vi "Set Alarm Colors and Get Alarm Text.vi"(9 "Alarm reference":refnum<vi>, 10 "Under Low Limit":bool, 11 "Over High Limit":bool) -> (3 "Alarm String":string)   [LabVIEW 2023]
doc: "Sets the colors of the Alarm display based on the alarm state and returns the text to display in the Alarm indicator."
uses:
  <vilib>/Utility/miscctls.llb/LVTextColorsTypeDef.ctl
panel:
  in  "Under Temp":string="UNDER TEMP"
  in  "Over Temp":string="OVER TEMP"
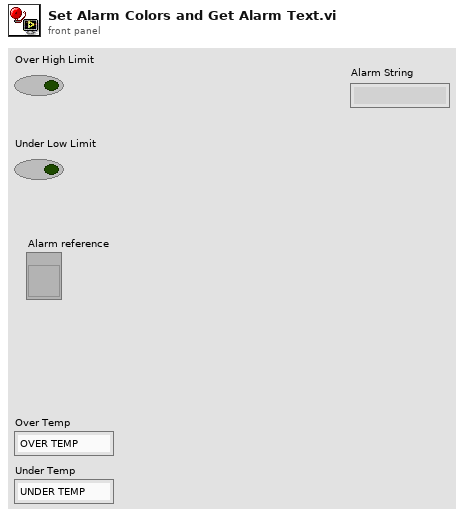
[diagram p1: front panel]
types:
  T1 = typedef "LVTextColorsTypeDef.ctl" = cluster{"Text Color":u32, "Background Color":u32}
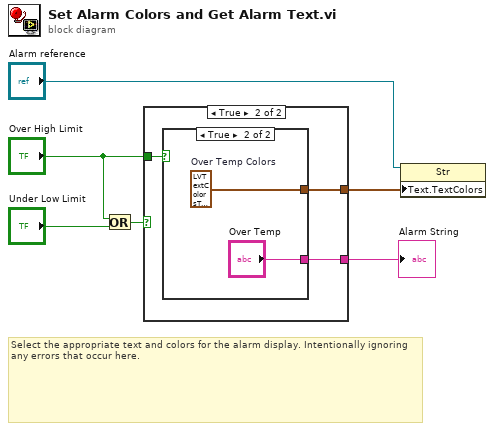
[diagram p0: block diagram]
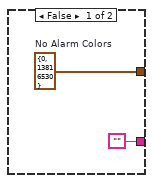
[diagram p2: hidden frame]
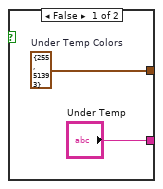
[diagram p3: hidden frame]
diagram:
  # "Select the appropriate text and colors for the alarm display. Intentionally ignoring any errors that occur here."
  n1 = Or(x="Over High Limit", y="Under Low Limit") -> (x .or. y?=w4:bool)
  n2 = case shown="True" w4 {
    tunnel: "Over High Limit" -> [_ w11]
    tunnel: [w8 w10] -> w2
    tunnel: ["" w9] -> w1
    frame False {
      w8 = T1 {"Text Color"=0, "Background Color"=13816530}  # No Alarm Colors
    }
    frame True {
      n3 = case shown="True" w11 {
        tunnel: [w13 w15] -> w10
        tunnel: ["Under Temp" "Over Temp"] -> w9
        frame False {
          w13 = T1 {"Text Color"=255, "Background Color"=51393}  # Under Temp Colors
        }
        frame True {
          w15 = T1 {"Text Color"=16449346, "Background Color"=11796481}  # Over Temp Colors
        }
      }
    }
  }
  "Alarm String" <- w1
  n4 = property class="Str"(reference="Alarm reference", "Text.TextColors"=w2) -> ()  [unwired: 1 in, 2 out]
